vi "empy_timestamp.vi"() -> (7 "empty time stamp":timestamp)   [LabVIEW 2015]
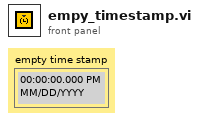
[diagram p1: front panel]
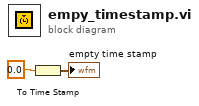
[diagram p0: block diagram]
diagram:
  n1 = To Time Stamp(1:0.0) -> (0:→"empty time stamp":timestamp)
